vi "New_lc.vi"(8 "error in (no error)":errorcluster caption="错误输入（无错误）", 10 "PictureRef":refnum<vi>, 11 "Picture_Class 输入":refnum<class "Picture_Class.lvclass"> caption="DNL_LabVIEW Object in") -> (0 "error out":errorcluster caption="错误输出", 3 "Picture_Class 输出":refnum<class "Picture_Class.lvclass"> caption="DNL_LabVIEW Object out")   [LabVIEW 2013, in "Picture_Class.lvclass"]
uses:
  Picture_Class.lvclass
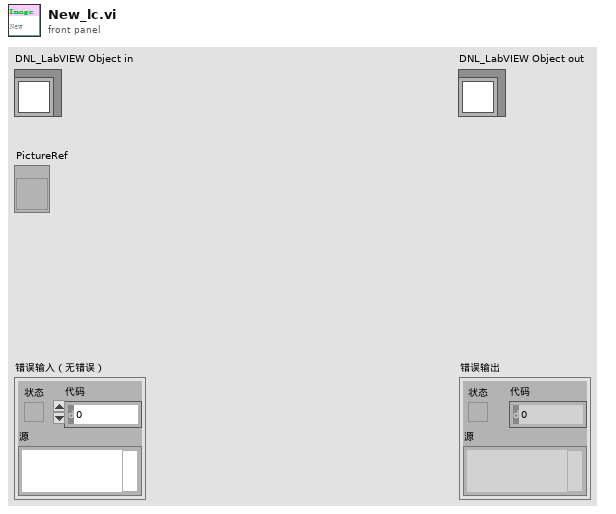
[diagram p1: front panel]
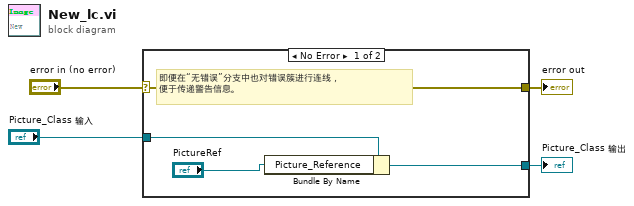
[diagram p0: block diagram]
diagram:
  n1 = case shown="No Error" "error in (no error)" {
    selector: "error in (no error)" -> [w8 w10]
    tunnel: [w8 w10] -> w3
    tunnel: [w6 w9] -> w1
    tunnel: "Picture_Class 输入" -> [w7 w9]
    frame No Error {
      # "即便在“无错误”分支中也对错误簇进行连线，\n便于传递警告信息。"
      n2 = Bundle By Name(cluster=w7, "Picture_Reference"="PictureRef") -> (w6:refnum<class "Picture_Class.lvclass">)
    }
    frame Error {
    }
  }
  "error out" <- w3
  "Picture_Class 输出" <- w1
